vi "Add Node.vi"(8 "error in (no error)":errorcluster, 9 "Parent":string, 10 "UID":string, 11 "Base Tree in":refnum<class "Base Tree.lvclass">) -> (0 "error out":errorcluster, 3 "Base Tree out":refnum<class "Base Tree.lvclass">)   [LabVIEW 2017, in "Browser Core.lvlib" / "Base Tree.lvclass"]
doc: "Create node with given UID and Add it as a child to the given Parent node. If the Parent input is empty, the node will be treated as a child of the Root Node."
uses:
  Base Tree.lvclass
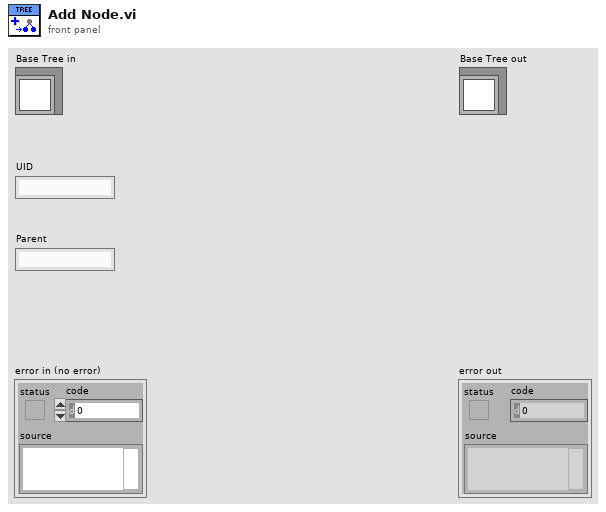
[diagram p1: front panel]
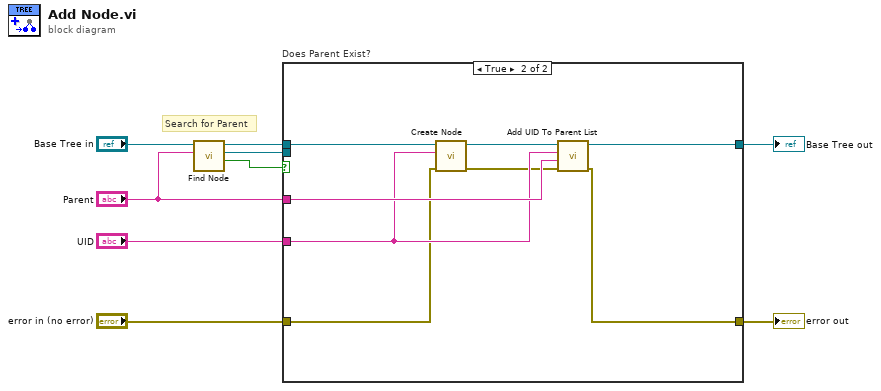
[diagram p0: block diagram]
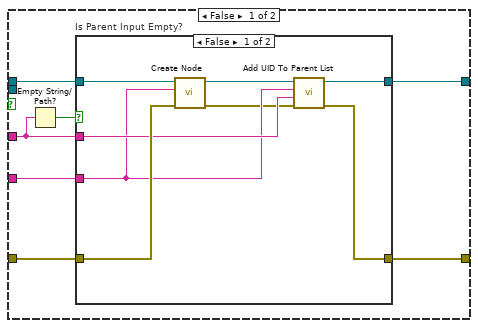
[diagram p2: hidden frame]
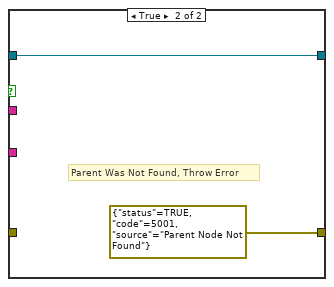
[diagram p3: hidden frame]
diagram:
  # "Search for Parent"
  n1 = call-dynamic "Find Node.vi"("UID"="Parent", "Base Tree in"="Base Tree in") -> ("Found?"=w4:bool, "Node"=w3:refnum<class "Generic Node.lvclass">, "Base Tree out"=w5:refnum<class "Base Tree.lvclass">)  [unwired: 5 in, 2 out]
  n2 = case "Does Parent Exist?" shown="True" w4 {
    tunnel: "error in (no error)" -> [w12 w29]
    tunnel: [w16 w27] -> w7
    tunnel: [w14 w32] -> w6
    tunnel: w5 -> [w15 w34]
    tunnel: w3 -> [_ _]
    tunnel: "UID" -> [w11 w30]
    tunnel: "Parent" -> [w10 w31]
    frame False {
      n3 = Empty String/Path?(string/path=w10) -> (empty?=w13:bool)
      n4 = case "Is Parent Input Empty?" shown="False" w13 {
        tunnel: [w17 errorcluster {"status"=TRUE, "code"=5001, "source"="Parent Node Not Found"} ("error in (no error)")] -> w16
        tunnel: w15 -> [w24 w25]
        tunnel: [w21 w25] -> w14
        tunnel: w12 -> [w23 _]
        tunnel: w11 -> [w19 _]
        tunnel: w10 -> [w20 _]
        frame False {
          n5 = call "Create Node.vi"("error in (no error)"=w23, "UID"=w19, "Base Tree in"=w24) -> ("error out"=w18:errorcluster, "Base Tree out"=w22:refnum<class "Base Tree.lvclass">)  [unwired: 7 in]
          n6 = call "Add UID To Parent List.vi"("Base Tree in"=w22, "UID"=w19, "Parent"=w20, "error in (no error)"=w18) -> ("Base Tree out"=w21:refnum<class "Base Tree.lvclass">, "error out"=w17:errorcluster)  [unwired: 5 in]
        }
        frame True {
          # "Parent Was Not Found, Throw Error"
        }
      }
    }
    frame True {
      n7 = call "Create Node.vi"("error in (no error)"=w29, "UID"=w30, "Base Tree in"=w34) -> ("error out"=w28:errorcluster, "Base Tree out"=w33:refnum<class "Base Tree.lvclass">)  [unwired: 7 in]
      n8 = call "Add UID To Parent List.vi"("Base Tree in"=w33, "UID"=w30, "Parent"=w31, "error in (no error)"=w28) -> ("Base Tree out"=w32:refnum<class "Base Tree.lvclass">, "error out"=w27:errorcluster)  [unwired: 5 in]
    }
  }
  "error out" <- w7
  "Base Tree out" <- w6
